vi "Get steps.vi"(8 "error in (no error)":errorcluster, 11 "Tomo in":refnum<class "Tomo.lvclass">) -> (0 "error out":errorcluster, 1 "Y step size":dbl[unit], 2 "X step size":dbl[unit], 3 "Tomo out":refnum<class "Tomo.lvclass">, 4 "Z step size":dbl[unit], 5 "number of views":dbl)   [LabVIEW 2012, in "Tomo.lvclass"]
uses:
  Tomo.lvclass
  Tomo.lvclass/Tomo.ctl
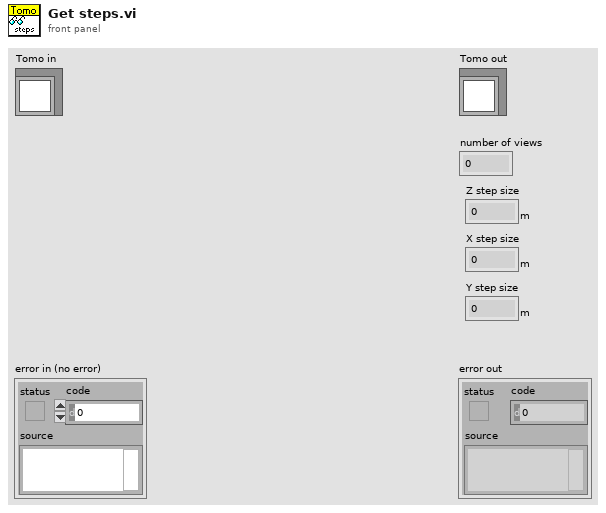
[diagram p1: front panel]
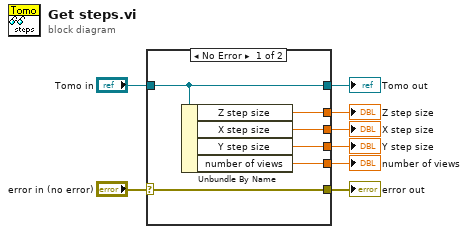
[diagram p0: block diagram]
diagram:
  n1 = case shown="No Error" "error in (no error)" {
    selector: "error in (no error)" -> [w14 w16]
    tunnel: [w14 w16] -> w7
    tunnel: [w13 w15] -> w5
    tunnel: "Tomo in" -> [w13 w15]
    tunnel: [w12 _] -> w4
    tunnel: [w11 _] -> w3
    tunnel: [w10 _] -> w2
    tunnel: [w9 _] -> w1
    frame No Error {
      n2 = Unbundle By Name(w13) -> ("Z step size"=w12:dbl[unit], "X step size"=w11:dbl[unit], "Y step size"=w10:dbl[unit], "number of views"=w9:dbl)
    }
    frame Error {
    }
  }
  "error out" <- w7
  "Tomo out" <- w5
  "Z step size" <- w4
  "X step size" <- w3
  "Y step size" <- w2
  "number of views" <- w1
